vi "reshape array (Ballard-1553-hw).vi"(10 "size requested":i32, 11 "hw configuration in":T1[](array[typedef])) -> (3 "hw configuration out":T1[](array[typedef]))   [LabVIEW 2020]
uses:
  1553/_controls/ballard1553_hw_map.ctl
  1553/_controls/ballard1553_RT_list.ctl
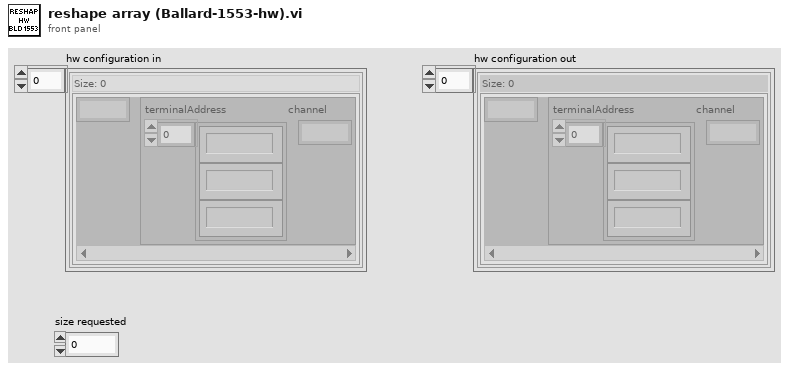
[diagram p1: front panel]
types:
  T1 = typedef "ballard1553_hw_map.ctl" = map{i32, T2}
  T2 = typedef "ballard1553_RT_list.ctl" = cluster{"terminalAddress":i32[], "channel":i32}
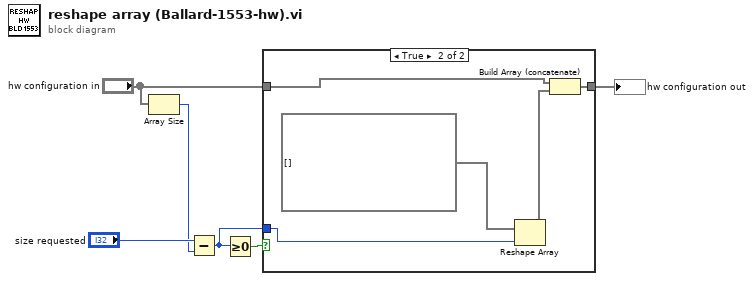
[diagram p0: block diagram]
diagram:
  n1 = Array Size(array="hw configuration in") -> (size(s)=w5:i32)
  n2 = Subtract(x="size requested", y=w5) -> (x-y=w3:i32)
  n3 = Greater Or Equal To 0?(x=w3) -> (x >= 0?=w4:bool)
  n4 = case shown="True" w4 {
    tunnel: w3 -> [_ w12]
    tunnel: "hw configuration in" -> [w7 w10]
    tunnel: [w7 w9] -> w1
    frame False {
    }
    frame True {
      n5 = Reshape Array(T1[] [] ("hw configuration"), w12) -> (w11:T1[])
      n6 = Build Array (concatenate)(w10, w11) -> (w9:T1[])
    }
  }
  "hw configuration out" <- w1
